vi "读取数据处理 (子VI).vi"(5 "data out":string) -> (3 "系统编码ST":string, 4 "CHECK?":bool, 6 "命令编码CN":string, 8 "设备编码MN":string, 10 "密码PW":string, 12 "数据":string, 14 "拆分包及应答Flag":string, 15 "时间QN":string)   [LabVIEW 2016, in "数据传输系统-02.lvlib"]
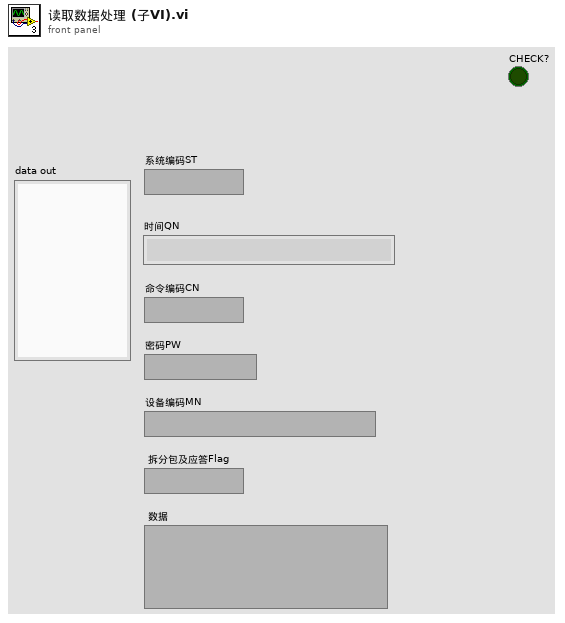
[diagram p1: front panel]
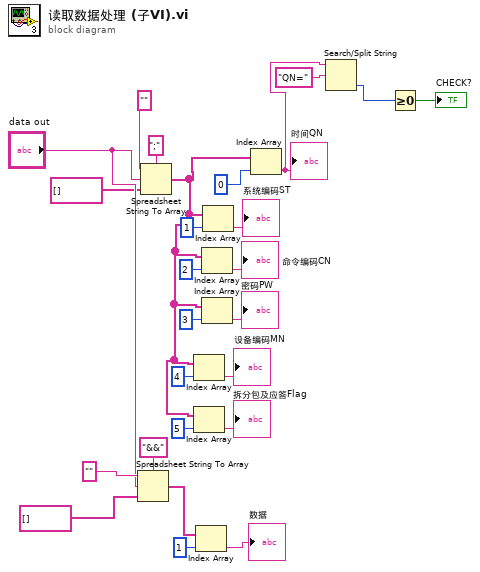
[diagram p0: block diagram]
diagram:
  n1 = Spreadsheet String To Array(delimiter (Tab)="&&" ("分隔符(Tab)"), format string="" ("格式字符串"), spreadsheet string="data out", array type (2D Dbl)=string[] [] ("数组")) -> (array=w24:string[])
  n2 = Spreadsheet String To Array(delimiter (Tab)=";" ("分隔符(Tab)"), format string="" ("格式字符串"), spreadsheet string="data out", array type (2D Dbl)=string[] [] ("数组")) -> (array=w8:string[])
  n3 = Index Array(array=w8, index=4 ("索引")) -> (element=→"设备编码MN":string)
  n4 = Index Array(array=w8, index=5 ("索引")) -> (element=→"拆分包及应答Flag":string)
  n5 = Index Array(array=w24, index=1 ("索引")) -> (element=→"数据":string)
  n6 = Index Array(array=w8, index=2 ("索引")) -> (element=→"命令编码CN":string)
  n7 = Index Array(array=w8, index=3 ("索引")) -> (element=→"密码PW":string)
  n8 = Index Array(array=w8, index=1 ("索引")) -> (element=→"系统编码ST":string)
  n9 = Index Array(array=w8, index=0 ("索引")) -> (element=w3:string)
  "时间QN" <- w3
  n10 = Search/Split String(string=w3, search string/char (-)="QN=" ("搜索字符串/字符(-)")) -> (offset of match=w2:i32)  [unwired: 1 in, 2 out]
  n11 = Greater Or Equal To 0?(x=w2) -> (x >= 0?=→"CHECK?":bool)
